vi "Toggle Selection.vi"(8 "error in (no error)":errorcluster, 10 "Tag":string, 11 "TreeSelectionSingle in":refnum<class "TreeSelectionSingle.lvclass">) -> (0 "error out":errorcluster, 3 "TreeSelectionSingle out":refnum<class "TreeSelectionSingle.lvclass">)   [LabVIEW 2015, in "TreeSelectionSingle.lvclass"]
doc: "<b> </b> <b> </b>\n©2016 Q Software Innovations, LLC (QSI)\nwritten by Quentin Alldredge\nproduced in LabVIEW 2015\n\nsupport@qsoftwareinnovations.com\nwww.qsoftwareinnovations.com\n\nAll rights reserved.\n\nRedistribution and use in source and binary forms, with or without modification, are permitted provided that the following conditions are met:\n\n * Redistributions of source code must retain the above copyright notice, this list of conditions and the following disclaimer.\n * Redistributions in binary form must reproduce the above copyright notice, this list of conditions and the following disclaimer in the documentation and/or other materials provided with the distribution.\n * Neither the name of Q Software Innovations, LLC. nor the names of its contributors may be used to endorse or promote products derived from this software without specific prior written permission.\n\nTHIS SOFTWARE IS PROVIDED BY THE COPYRIGHT HOLDERS AND CONTRIBUTORS \"AS IS\" AND ANY EXPRESS OR IMPLIED WARRANTIES, INCLUDING, BUT NOT LIMITED TO, THE IMPLIED WARRANTIES OF MERCHANTABILITY AND FITNESS FOR A PARTICULAR PURPOSE ARE DISCLAIMED. IN NO EVENT SHALL THE COPYRIGHT OWNER OR CONTRIBUTORS BE LIABLE FOR ANY DIRECT, INDIRECT, INCIDENTAL, SPECIAL, EXEMPLARY, OR CONSEQUENTIAL DAMAGES (INCLUDING, BUT NOT LIMITED TO, PROCUREMENT OF SUBSTITUTE GOODS OR SERVICES; LOSS OF USE, DATA, OR PROFITS; OR BUSINESS INTERRUPTION) HOWEVER CAUSED AND ON ANY THEORY OF LIABILITY, WHETHER IN CONTRACT, STRICT LIABILITY, OR TORT (INCLUDING NEGLIGENCE OR OTHERWISE) ARISING IN ANY WAY OUT OF THE USE OF THIS SOFTWARE, EVEN IF ADVISED OF THE POSSIBILITY OF SUCH DAMAGE."
uses:
  TreeSelectionSingle.lvclass
  TreeSelection/TreeSelection.lvclass
  TreeControl/TreeControl.lvclass
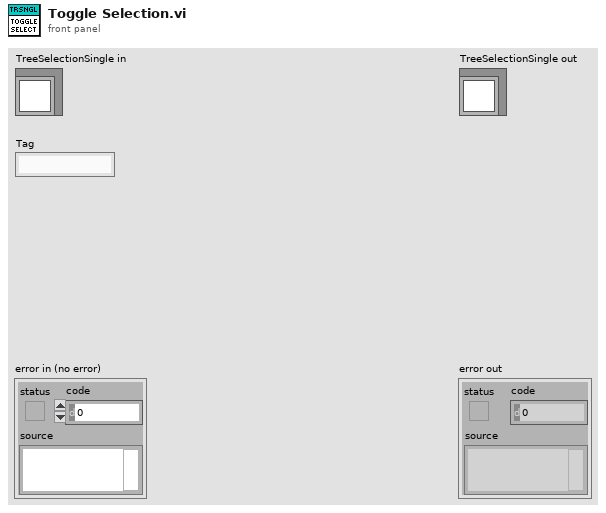
[diagram p1: front panel]
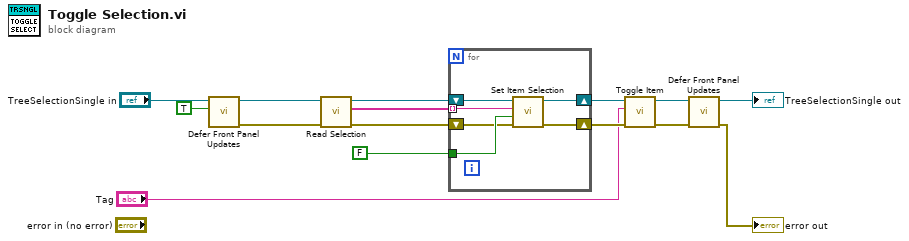
[diagram p0: block diagram]
diagram:
  n1 = call "Defer Front Panel Updates.vi"("Defer Panel Updates (F)"=TRUE, "Tree in"="TreeSelectionSingle in") -> ("error out"=w5:errorcluster, "Tree (dup)"=w9:refnum<class "TreeSelectionSingle.lvclass">)  [unwired: 8 in]
  n2 = call-dynamic "Read Selection.vi"("error in (no error)"=w5, "TreeSelection in"=w9) -> ("error out"=w6:errorcluster, "Selection[]"=w7:string[], "TreeSelection out"=w8:refnum<class "TreeSelectionSingle.lvclass">)  [unwired: 7 in]
  n3 = for {
    tunnel: w7 -> [w20] mode=indexing
    shift-right: [w19] -> w14
    shift-left: w8 -> [w21]
    tunnel: FALSE -> [w18]
    shift-right: [w16] -> w4
    shift-left: w6 -> [w17]
    n4 = call-dynamic "Set Item Selection.vi"("error in (no error)"=w17, "Selected?"=w18, "Tag"=w20, "TreeSelection in"=w21) -> ("error out"=w16:errorcluster, "TreeSelection out"=w19:refnum<class "TreeSelectionSingle.lvclass">)  [unwired: 6 in]
  }
  n5 = call "Toggle Item.vi"("error in (no error)"=w4, "Tag"="Tag", "TreeSelection in"=w14) -> ("error out"=w3:errorcluster, "TreeSelection out"=w11:refnum<class "TreeSelectionSingle.lvclass">)  [unwired: 7 in]
  n6 = call "Defer Front Panel Updates.vi"("error in (no error)"=w3, "Tree in"=w11) -> ("error out"=→"error out":errorcluster, "Tree (dup)"=→"TreeSelectionSingle out":refnum<class "TreeSelectionSingle.lvclass">)  [unwired: 8 in]
